vi "Close MeasurementLink Session.vi"(8 "error in":errorcluster, 9 "initialize and close session behavior":T1, 10 "session in":variant, 11 "instrument in":refnum<class "Instrument.lvclass">) -> (0 "error out":errorcluster)   [LabVIEW 2020, in "MeasurementLink niScope.lvlib" / "Instrument.lvclass"]
uses:
  Instrument.lvclass
  MeasurementLink Instrument/IInstrument/Initialize and Close Session Behavior.ctl
  MeasurementLink Measurement Server/Helpers/Error Strings Global Internal.vi
  MeasurementLink Instrument/IInstrument/IInstrument.lvclass
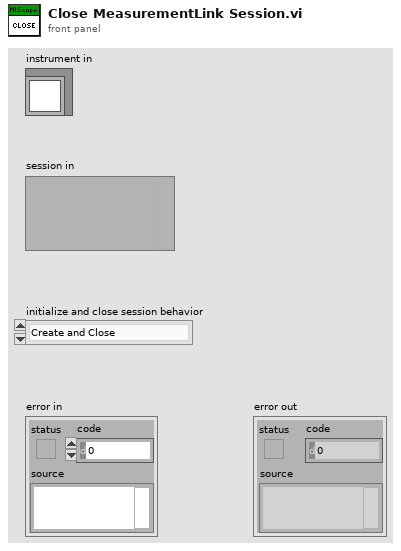
[diagram p1: front panel]
types:
  T1 = typedef "MeasurementLink Instrument.lvlib/IInstrument.lvclass/Initialize and Close Session Behavior.ctl" = enum16{"Create and Close", "Attach and Detach", "Create and Detach", "Attach and Close"}
  T2 = typedef "MeasurementLink Instrument.lvlib/IInstrument.lvclass/Close Session Behavior.ctl" = enum16{"Close Session", "Detach Session"}
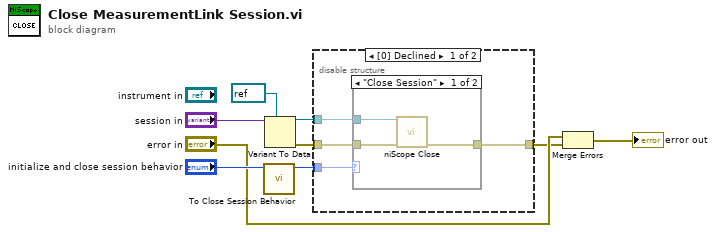
[diagram p0: block diagram]
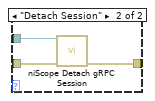
[diagram p2: hidden frame]
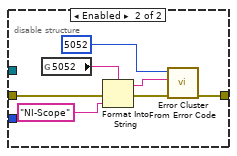
[diagram p3: hidden frame]
diagram:
  n1 = call "To Close Session Behavior.vi"("initialize and close session behavior"="initialize and close session behavior") -> ("close session behavior"=w1:T2)  [unwired: 10 in]
  n2 = Variant To Data(type=refnum<k15> refnum ("instrument handle"), Variant="session in") -> (data=w3:refnum<k15>, error out=w8:errorcluster)  [unwired: 1 in]
  n3 = disable-structure shown="[0] Declined" {
    disable-tunnel: w1 -> [w13 _]
    disable-tunnel: w8 -> [w12 w20]
    disable-tunnel: [w11 w26] -> w5
    disable-tunnel: w3 -> [w10 _]
    frame Disabled {
      n4 = case shown="\"Close Session\"" w13 {
        tunnel: w12 -> [w16 w19]
        tunnel: [w15 w18] -> w11
        tunnel: w10 -> [w14 w17]
        frame "Close Session" {
          n5 = call <instrlib>:"niScope Close.vi"("instrument handle"=w14, "error in"=w16) -> ("error out"=w15:errorcluster)  [unwired: 13 in]
        }
        frame "Detach Session" {
          n6 = call <instrlib>:"niScope Detach gRPC Session.vi"("instrument handle"=w17, "error in"=w19) -> ("error out"=w18:errorcluster)  [unwired: 13 in]
        }
      }
    }
    frame Enabled {
      n7 = global read "Error Strings Global Internal.vi" "5052"() -> (w24:string)
      n8 = Format Into String(format string=w24, error in=w20, "NI-Scope") -> (resulting string=w21:string, error out=w22:errorcluster)  [unwired: 1 in]
      n9 = call <vilib>:"Error Cluster From Error Code.vi"("error in (no error)"=w22, "error message (\"\")"=w21, "error code (0)"=5052) -> ("error out"=w26:errorcluster)  [unwired: 6 in]
    }
  }
  n10 = Merge Errors("error in", w5) -> (→"error out":errorcluster)
